vi "Rinocloud_global_variable.vi"() -> ()   [LabVIEW 2011, in "Rinocloud Library.lvlib"]
uses:
  Rinocloud Library.lvlib
panel:
  in  "Active item name":string="<folder> home (id=)"
  in  "Active directory ID":string
  in  "Active file ID":string
  in  "Active object ID":string
  in  "Rino url":string="https://rinocloud.com/api/1/files/"
  in  "Tab Control":enum32{"Communication"}(tab)
  in  "Token":string
  in  "Local storage root path":path=path "C:/Rinocloud mirror"
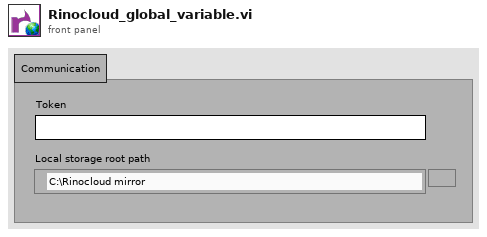
[diagram p1: front panel]
diagram:
